vi "test.vi"() -> ()   [LabVIEW 2012]
panel:
  out "二维图片":picture
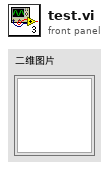
[diagram p1: front panel]
types:
  T1 = typedef "imagedata.ctl" = cluster{"image type":i32, "image depth":i32, "image":u8[], "mask":u8[], "colors":u32[], "Rectangle":cluster{"left":i16, "top":i16, "right":i16, "bottom":i16}}
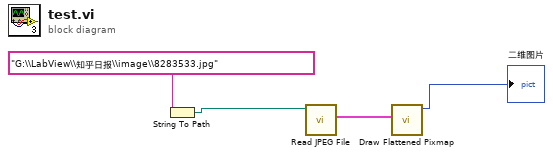
[diagram p0: block diagram]
diagram:
  n1 = String To Path(string="G:\\LabView\\知乎日报\\image\\8283533.jpg") -> (path=w3:path)
  n2 = call <vilib>:"Read JPEG File.vi"("path to JPEG file"=w3) -> ("image data"=w2:T1)  [unwired: 8 in, 2 out]
  n3 = call <vilib>:"Draw Flattened Pixmap.vi"("image data"=w2) -> ("new picture"=→"二维图片":picture)  [unwired: 8 in]
